vi "calculateCRC.vi"(8 "error in (no error)":errorcluster, 10 "Length":u16, 11 "ModbusBuffer in":refnum<class "ModbusBufferBuilder.lvclass">) -> (0 "error out":errorcluster, 2 "CRC":u16, 3 "ModbusBuffer out":refnum<class "ModbusBufferBuilder.lvclass">)   [LabVIEW 2016, in "ModbusBufferBuilder.lvclass"]
uses:
  ModbusBufferBuilder.lvclass
  ModbusBufferBuilder.lvclass/ModbusBufferBuilder.ctl
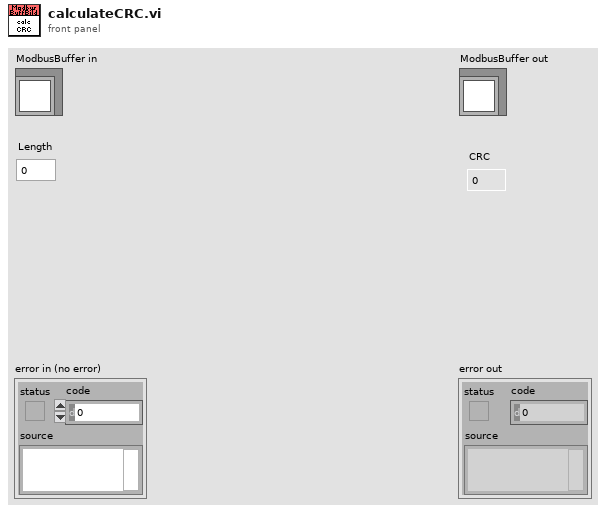
[diagram p1: front panel]
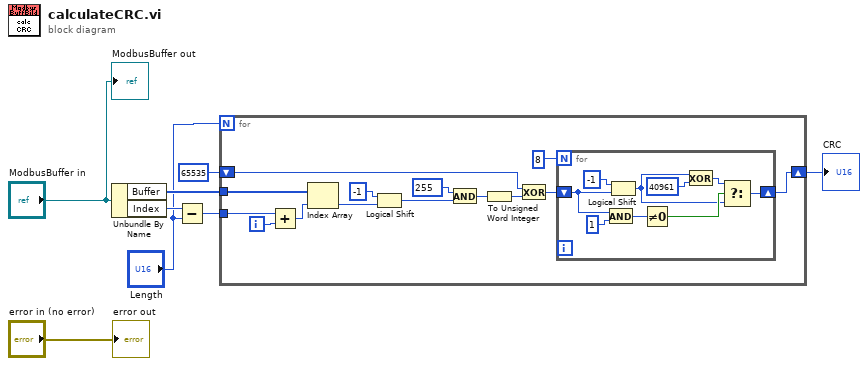
[diagram p0: block diagram]
diagram:
  n1 = Unbundle By Name("ModbusBuffer in") -> ("Buffer"=w6:u16[], "Index"=w3:i32)
  n2 = Subtract(x=w3, y="Length") -> (x-y=w5:i32)
  n3 = for {
    N: "Length" -> [_]
    tunnel: w6 -> [w17]
    shift-right: [w19] -> w1
    shift-left: u16 65535 -> [w21]
    tunnel: w5 -> [w15]
    i -> [w16]
    n4 = Add(x=w15, y=w16) -> (x+y=w14:i32)
    n5 = Index Array(array=w17, index=w14) -> (element=w13:u16)
    n6 = Logical Shift(y=i16 -1, x=w13) -> (x << y=w11:u16)
    n7 = And(x=u16 255, y=w11) -> (x .and. y?=w9:u16)
    n8 = To Unsigned Word Integer(number=w9) -> (unsigned 16bit integer=w18:u16)
    n9 = Exclusive Or(1:w18, 2:w21) -> (0:w20:u16)
    n10 = for {
      N: 8 -> [_]
      shift-right: [w24] -> w19
      shift-left: w20 -> [w25]
      n11 = And(x=w25, y=u16 1) -> (x .and. y?=w31:u16)
      n12 = Logical Shift(y=i16 -1, x=w25) -> (x << y=w23:u16)
      n13 = Not Equal To 0?(x=w31) -> (x != 0?=w30:bool)
      n14 = Exclusive Or(1:u16 40961 ("y"), 2:w23) -> (0:w26:u16)
      n15 = Select(t=w26, s=w30, f=w23) -> (s? t:f=w24:u16)
    }
  }
  "CRC" <- w1
  "error out" <- "error in (no error)"
  "ModbusBuffer out" <- "ModbusBuffer in"
